vi "Autotune.vi"(6 "PID Coeffs":cluster{"P1":dbl, "P2":dbl, "P3":dbl}, 7 "Parameters of Filter\n(PI > 0,7; PID > 1,7) in":dbl, 9 "Parameters of the control object W(p)":T1, 10 "Selecting the type of regulator  \nfor Ziegler–Nichols method":enum16{"PID", "PI", "P"}(ring), 11 "Settings Methods Panel":enum32{"Ziegler  -  Nichols", "IMC", "Amigo"}(ring)) -> (1 "P3":dbl, 2 "P2":dbl, 3 "P1":dbl, 4 "Parameters of Filter\n(PI > 0,7; PID > 1,7) out":dbl)   [LabVIEW 2014]
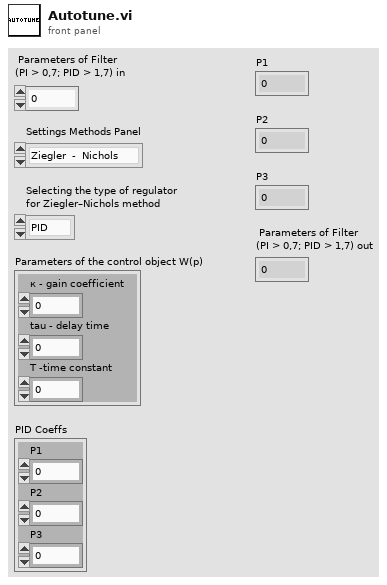
[diagram p1: front panel]
types:
  T1 = cluster{"к - gain coefficient":dbl, "tau - delay time":dbl, "T -time constant":dbl}
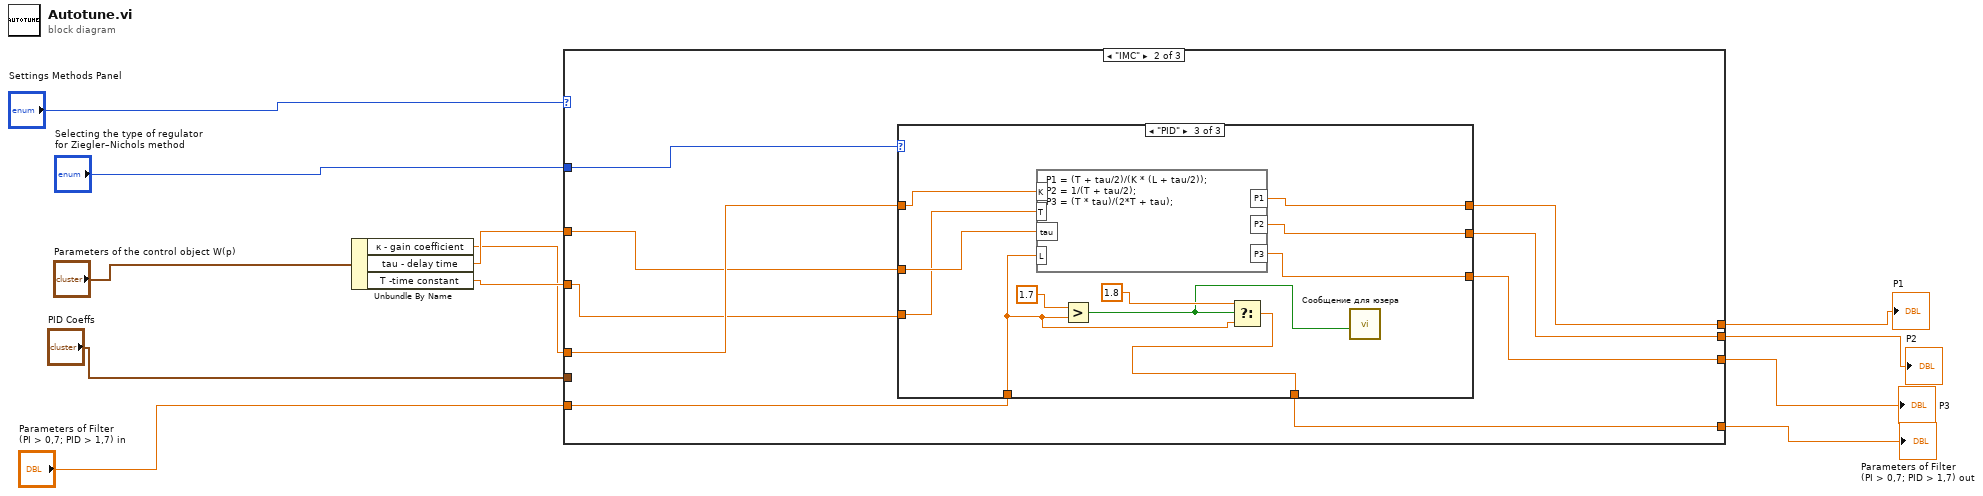
[diagram p0: block diagram]
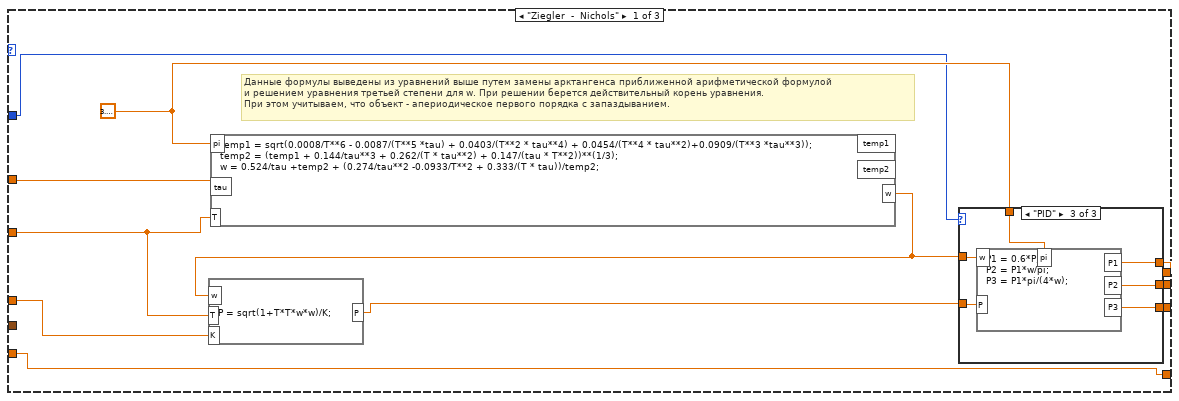
[diagram p2: hidden frame]
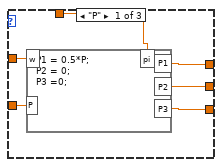
[diagram p3: hidden frame]
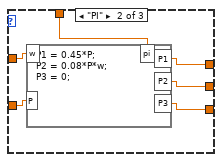
[diagram p4: hidden frame]
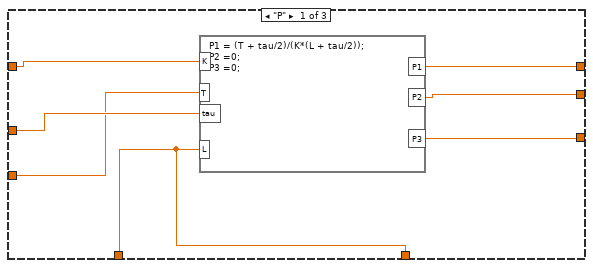
[diagram p5: hidden frame]
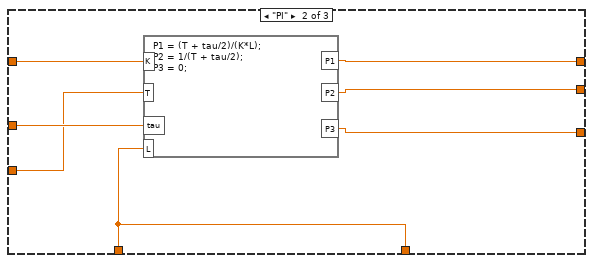
[diagram p6: hidden frame]
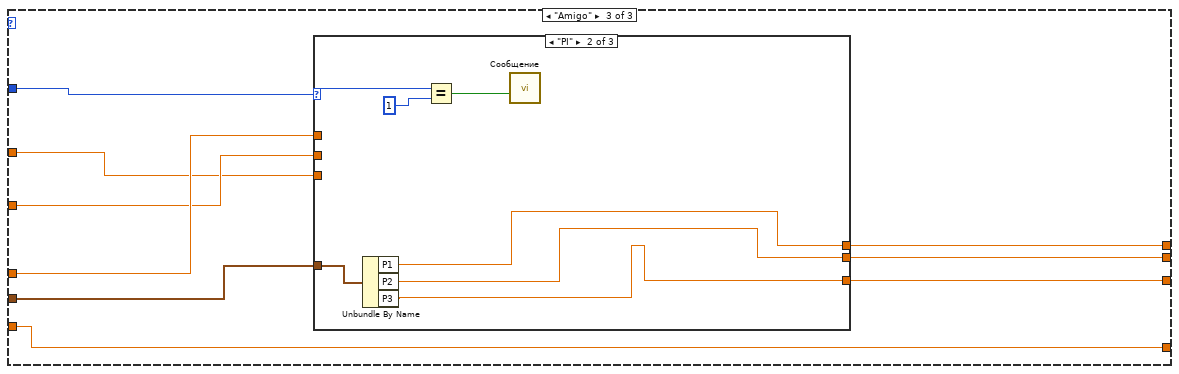
[diagram p7: hidden frame]
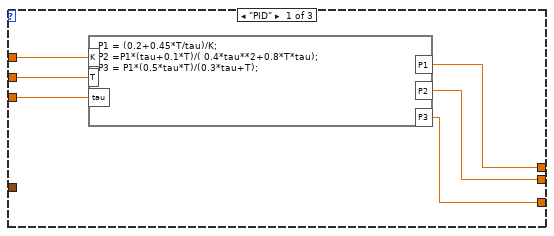
[diagram p8: hidden frame]
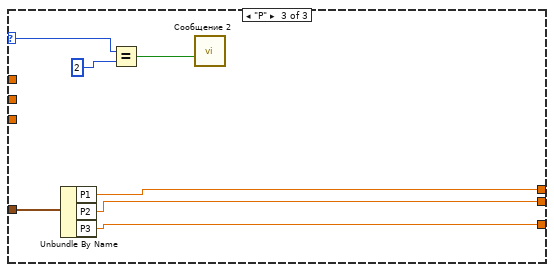
[diagram p9: hidden frame]
diagram:
  n1 = Unbundle By Name("Parameters of the control object W(p)") -> ("к - gain coefficient"=w2:dbl, "tau - delay time"=w3:dbl, "T -time constant"=w4:dbl)
  n2 = case shown="\"IMC\"" "Settings Methods Panel" {
    tunnel: w2 -> [w18 w50 w84]
    tunnel: w3 -> [w20 w49 w82]
    tunnel: w4 -> [w19 w48 w83]
    tunnel: [w17 w47 w81] -> w6
    tunnel: [w16 w46 w80] -> w7
    tunnel: [w15 w45 w79] -> w8
    tunnel: "Parameters of Filter\n(PI > 0,7; PID > 1,7) in" -> [w13 w44 w76]
    tunnel: "Selecting the type of regulator  \nfor Ziegler–Nichols method" -> [w14 w43 w78]
    tunnel: "PID Coeffs" -> [_ _ w77]
    tunnel: [w13 w42 w76] -> w12
    frame "Ziegler  -  Nichols" {
      w21 = 3.141592653589793
      # "Данные формулы выведены из уравнений выше путем замены арктангенса приближенной арифметической формулой\nи решением уравнения третьей степени для w. При решении берется действительный корень уравнения.\nПри этом учитываем, что объект - апериодическое первого порядка с запаздыванием."
      n3 = formula code="temp1 = sqrt(0.0008/T**6 - 0.0087/(T**5 *tau) + 0.0403/(T**2 * tau**4) + 0.0454/(T**4 * tau**2)+0.0909/(T**3 *tau**3));\ntemp2 = (temp1 + 0.144/tau**3 + 0.262/(T * tau**2) + 0.147/(tau * T**2))**(1/3);\nw = 0.524/tau +temp2 + (0.274/tau**2 -0.0933/T**2 + 0.333/(T * tau))/temp2;"("pi"=w21, "T"=w19, "tau"=w20) -> ("w"=w22:dbl)  [unwired: 2 out]
      n4 = formula code="P = sqrt(1+T*T*w*w)/K;"("w"=w22, "T"=w19, "K"=w18) -> ("P"=w23:dbl)
      n5 = case shown="\"PID\"" w14 {
        tunnel: w23 -> [w29 w34 w39]
        tunnel: w22 -> [w28 w35 w40]
        tunnel: w21 -> [w27 w33 w41]
        tunnel: [w26 w32 w38] -> w17
        tunnel: [w25 w31 w37] -> w16
        tunnel: [w24 w30 w36] -> w15
        frame "P" {
          n6 = formula code="P1 = 0.5*P;\nP2 = 0;\nP3 =0;"("w"=w28, "P"=w29, "pi"=w27) -> ("P1"=w26:dbl, "P2"=w25:dbl, "P3"=w24:dbl)
        }
        frame "PI" {
          n7 = formula code="P1 = 0.45*P;\nP2 = 0.08*P*w;\nP3 = 0;"("w"=w35, "P"=w34, "pi"=w33) -> ("P1"=w32:dbl, "P2"=w31:dbl, "P3"=w30:dbl)
        }
        frame "PID" {
          n8 = formula code="P1 = 0.6*P;\nP2 = P1*w/pi;\nP3 = P1*pi/(4*w);"("w"=w40, "P"=w39, "pi"=w41) -> ("P1"=w38:dbl, "P2"=w37:dbl, "P3"=w36:dbl)
        }
      }
    }
    frame "IMC" {
      n9 = case shown="\"PID\"" w43 {
        tunnel: w50 -> [w57 w64 w75]
        tunnel: w49 -> [w56 w63 w74]
        tunnel: w48 -> [w55 w62 w73]
        tunnel: w44 -> [w51 w58 w67]
        tunnel: [w54 w61 w72] -> w47
        tunnel: [w53 w60 w71] -> w46
        tunnel: [w52 w59 w70] -> w45
        tunnel: [w51 w58 w65] -> w42
        frame "P" {
          n10 = formula code="P1 = (T + tau/2)/(K*(L + tau/2));\nP2 =0;\nP3 =0;"("K"=w57, "T"=w55, "tau"=w56, "L"=w51) -> ("P1"=w54:dbl, "P2"=w53:dbl, "P3"=w52:dbl)
        }
        frame "PI" {
          n11 = formula code="P1 = (T + tau/2)/(K*L);\nP2 = 1/(T + tau/2);\nP3 = 0;"("K"=w64, "T"=w62, "tau"=w63, "L"=w58) -> ("P1"=w61:dbl, "P2"=w60:dbl, "P3"=w59:dbl)
        }
        frame "PID" {
          n12 = formula code="P1 = (T + tau/2)/(K * (L + tau/2));\nP2 = 1/(T + tau/2);\nP3 = (T * tau)/(2*T + tau);"("K"=w75, "T"=w73, "tau"=w74, "L"=w67) -> ("P1"=w72:dbl, "P2"=w71:dbl, "P3"=w70:dbl)
          n13 = Greater?(x=1.7, y=w67) -> (0:w66:bool)
          n14 = Select(t=1.8, s=w66, f=w67) -> (s? t:f=w65:dbl)
          n15 = call "Сообщение для юзера"("Enable"=w66) -> ()  [unwired: 9 in, 2 out]
        }
      }
    }
    frame "Amigo" {
      n16 = case shown="\"PI\"" w78 {
        selector: w78 -> [_ w96 w102]
        tunnel: w84 -> [w90 _ _]
        tunnel: w83 -> [w89 _ _]
        tunnel: w82 -> [w88 _ _]
        tunnel: [w87 w93 w100] -> w81
        tunnel: [w86 w92 w99] -> w80
        tunnel: [w85 w91 w98] -> w79
        tunnel: w77 -> [_ w94 w101]
        frame "PID" {
          n17 = formula code="P1 = (0.2+0.45*T/tau)/K;\nP2 =P1*(tau+0.1*T)/( 0.4*tau**2+0.8*T*tau);\nP3 = P1*(0.5*tau*T)/(0.3*tau+T);"("K"=w90, "T"=w89, "tau"=w88) -> ("P1"=w87:dbl, "P2"=w86:dbl, "P3"=w85:dbl)
        }
        frame "PI" {
          n18 = Unbundle By Name(w94) -> ("P1"=w93:dbl, "P2"=w92:dbl, "P3"=w91:dbl)
          n19 = Equal?(x=w96, y=1) -> (x = y?=w95:bool)
          n20 = call "Сообщение"("Enable"=w95) -> ()  [unwired: 9 in, 2 out]
        }
        frame "P" {
          n21 = Unbundle By Name(w101) -> ("P1"=w100:dbl, "P2"=w99:dbl, "P3"=w98:dbl)
          n22 = Equal?(x=w102, y=2) -> (x = y?=w103:bool)
          n23 = call "Сообщение 2"("Enable"=w103) -> ()  [unwired: 9 in, 2 out]
        }
      }
    }
  }
  "Parameters of Filter\n(PI > 0,7; PID > 1,7) out" <- w12
  "P3" <- w8
  "P2" <- w7
  "P1" <- w6
